vi "RUN VI.vi"(8 "error in (no error)":errorcluster, 10 "VI path":path) -> (0 "error out":errorcluster)   [LabVIEW 2017]
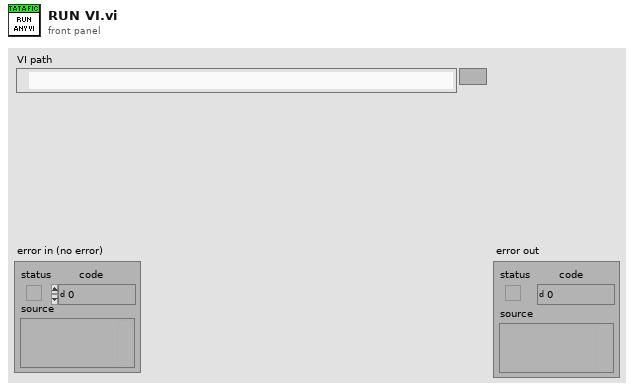
[diagram p1: front panel]
types:
  T1 = enum32{"Bad", "Idle", "Run top level", "Running"}
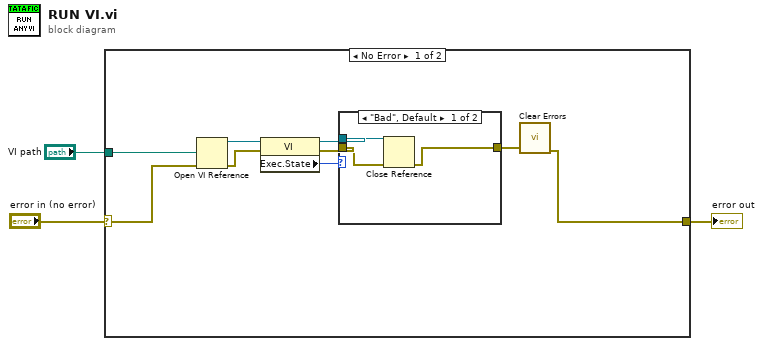
[diagram p0: block diagram]
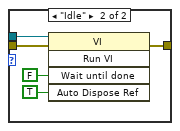
[diagram p2: hidden frame]
diagram:
  n1 = case shown="No Error" "error in (no error)" {
    selector: "error in (no error)" -> [w11 w21]
    tunnel: [w4 w21] -> w2
    tunnel: "VI path" -> [w12 _]
    frame No Error {
      n2 = Open VI Reference(vi path=w12, error in (no error)=w11) -> (vi reference=w10:refnum<vi>, error out=w9:errorcluster)  [unwired: 4 in]
      n3 = property class="VI"(reference=w10, error in=w9) -> (reference out=w8:refnum<vi>, error out=w7:errorcluster, "Exec.State"=w6:T1)
      n4 = case shown="\"Bad\", Default" w6 {
        tunnel: [w13 w18] -> w5
        tunnel: w7 -> [w14 w17]
        tunnel: w8 -> [w15 w16]
        frame "Bad", Default {
          n5 = Close Reference(reference=w15, error in (no error)=w14) -> (error out=w13:errorcluster)
        }
        frame "Idle" {
          n6 = invoke class="VI" method="Run VI"(reference=w16, error in=w17, "Wait until done"=FALSE ("Wait Until Done"), "Auto Dispose Ref"=TRUE ("Auto Dispose Reference")) -> (error out=w18:errorcluster)  [unwired: 1 in, 4 out]
        }
      }
      n7 = call <vilib>:"Clear Errors.vi"("error in (no error)"=w5) -> ("error out"=w4:errorcluster)  [unwired: 5 in, 1 out]
    }
    frame Error {
    }
  }
  "error out" <- w2
